vi "Monitornew new.vi"() -> ()   [LabVIEW 2019]
uses:
  <vilib>/Utility/file.llb/Write Delimited Spreadsheet (string).vi
  <userlib>/LevyLab/LV to ITX/Main/LV to DAT 1D.vi
panel:
  in  "shunt resistor":dbl=100000.0 format="%#_13g"
  in  "Tab Control":enum32{"Conductance"}(tab)
  in  "Voltage Pairs (+, -,...)":i32[][](array[numeric])=[[0, 0, 1, 2], [6, 6, 4, 3]]
  in  "Current (I-)":i32=3
  out "Two Terminal Conductance":cluster{"Y":dbl[], "Y":dbl[]}[](graph) caption="XY Graph"
  out "Four Terminal Resistance":cluster{"Y":dbl[], "Y":dbl[]}[](graph) caption="XY Graph"
  in  "Excitation voltage":dbl=0.1
  in  "Reset":bool
  out "Four Terminal conductance":cluster{"Y":dbl[], "Y":dbl[]}[](graph) caption="XY Graph"
  in  "wait (ms)":u32=60
  out "Humidity":dbl
  out "Temperature":dbl
  in  "error in (no error)":errorcluster
  in  "stop":bool
  in  "filename":string="test"
  in  "base path":path=path "G:/My Drive/ansom/Data/MFP3D/Test Files/monitor"
  in  "Comments":string
  in  "folder name":string="monitor"
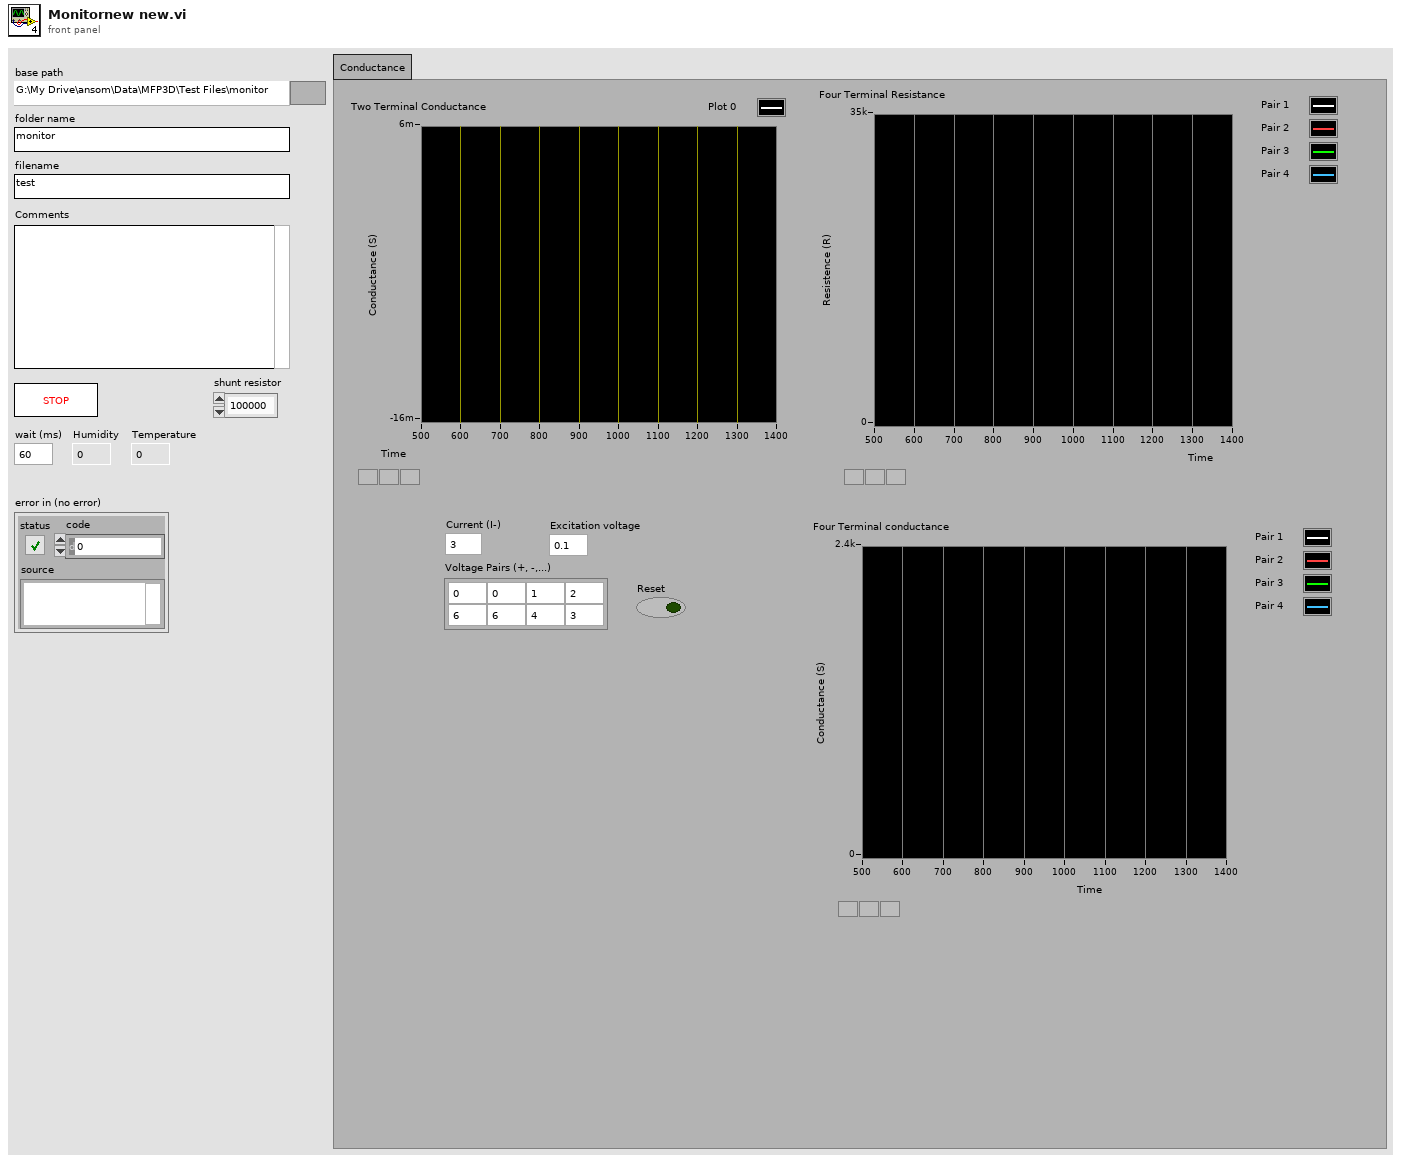
[diagram p1: front panel]
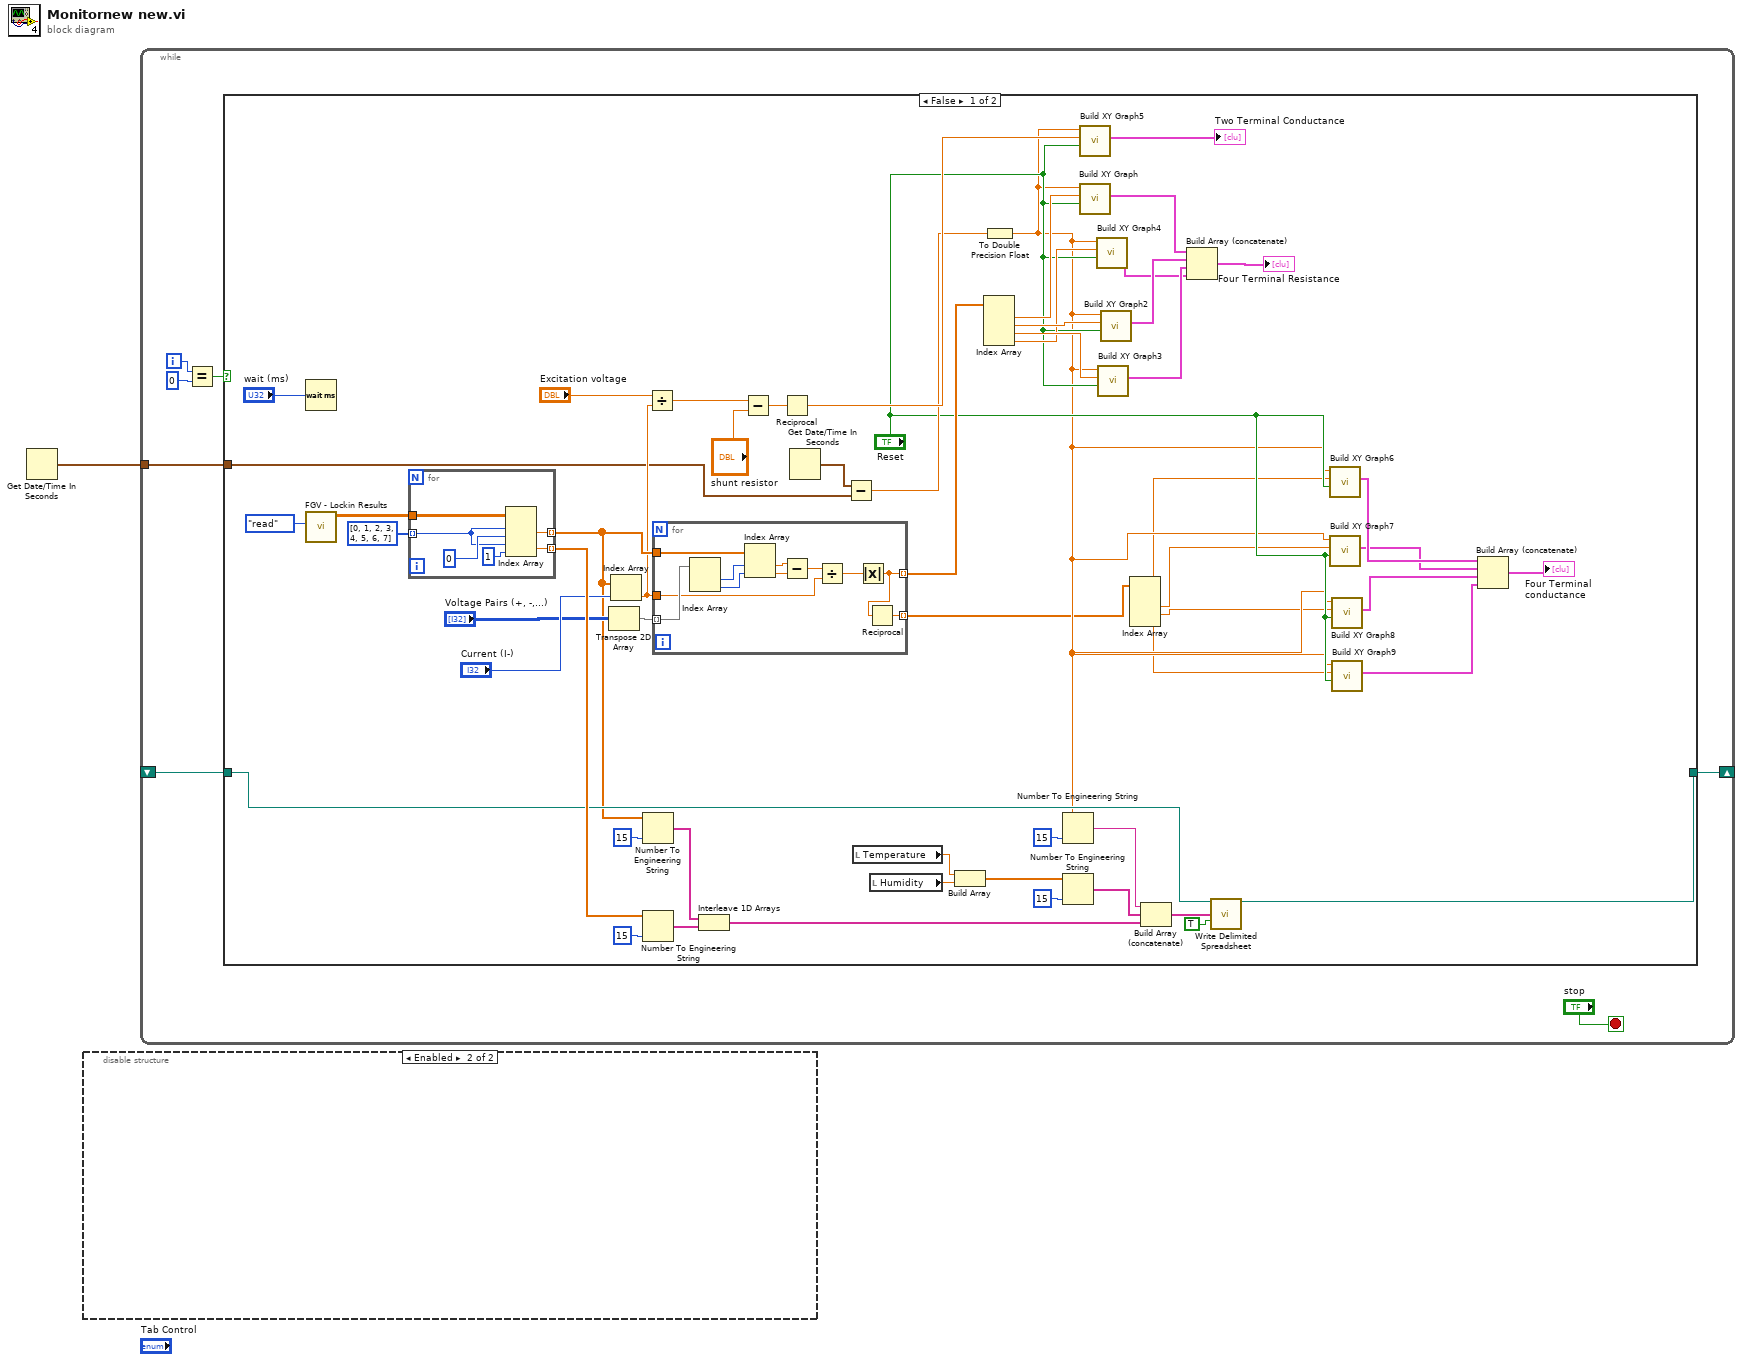
[diagram p0: block diagram]
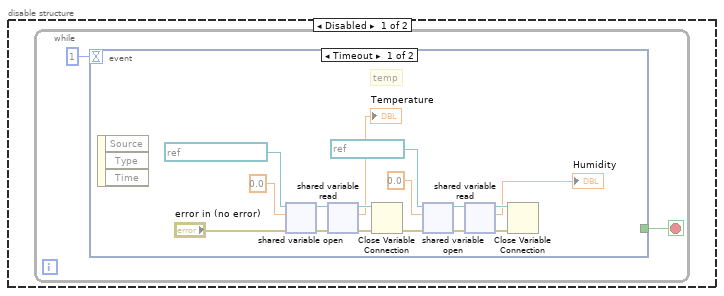
[diagram p2: hidden frame]
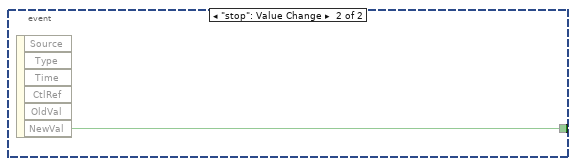
[diagram p3: hidden frame]
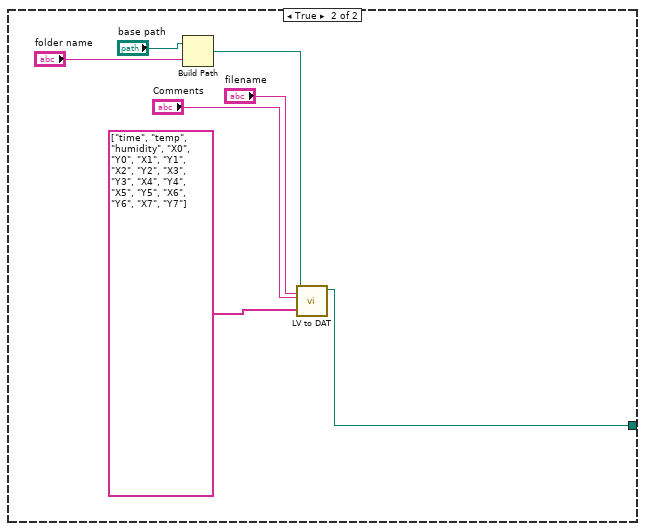
[diagram p4: hidden frame]
diagram:
  n1 = Get Date/Time In Seconds() -> (seconds since 1Jan1904=w1:timestamp)
  n2 = disable-structure shown="Enabled" {
    frame Disabled {
      n3 = while {
        stop <- w3 stop-if-true
        n4 = event shown="[0] Timeout" {
          selector: _ -> [_ _]
          dyn-events: _ -> [_ _]
          timeout: 1 -> [_ _]
          tunnel: [_ w20] -> w3
          event Timeout {
            # "temp"
            n5 = event-data() -> ()  [unwired: 1 in, 3 out]
            n6 = shared-variable-open(refnum<k21> "ni.var.psp://housesoftheholy/MFP3D/MFP3D Temperature" ("shared variable refnum in"), "error in (no error)", 0.0 ("Excitation voltage 2")) -> (w19:refnum<k21>, w18:errorcluster)  [unwired: 1 in]
            n7 = shared-variable-read(w19, w18) -> (w13:refnum<k21>, w12:errorcluster, →"Temperature":dbl)  [unwired: 1 out]
            n8 = Close Variable Connection(8:w12, 11:w13) -> (0:w6:errorcluster)
            n9 = shared-variable-open(refnum<k21> "ni.var.psp://housesoftheholy/MFP3D/MFP3D Hum" ("shared variable refnum in"), w6, 0.0 ("Excitation voltage 2")) -> (w16:refnum<k21>, w15:errorcluster)  [unwired: 1 in]
            n10 = shared-variable-read(w16, w15) -> (w11:refnum<k21>, w10:errorcluster, →"Humidity":dbl)  [unwired: 1 out]
            n11 = Close Variable Connection(8:w10, 11:w11) -> ()  [unwired: 1 out]
          }
          event "stop": Value Change {
            n12 = event-data() -> ("NewVal"=w20:bool)  [unwired: 1 in, 5 out]
          }
        }
      }
    }
    frame Enabled {
    }
  }
  n13 = while {
    shift-right: [w23] -> _
    shift-left: _ -> [w22]
    tunnel: w1 -> [w21]
    i -> [w27]
    stop <- "stop" stop-if-true
    n14 = Equal?(x=w27, y=0) -> (x = y?=w25:bool)
    n15 = case shown="False" w25 {
      tunnel: [w72 w102] -> w23
      tunnel: w22 -> [w75 _]
      tunnel: w21 -> [w48 _]
      frame False {
        n16 = Wait (ms)(milliseconds to wait="wait (ms)") -> ()  [unwired: 1 out]
        n17 = call <userlib>:"FGV - Lockin Results.vi"("Function"=enum16{"write", "read"}."read") -> ("Input Signals"=w82:dbl[][])  [unwired: 5 in, 1 out]
        n18 = for {
          tunnel: w82 -> [w98]
          tunnel: i32[] [0, 1, 2, 3, 4, 5, 6, 7] ("Lockins") -> [w99] mode=indexing
          tunnel: [w96] -> w60 mode=indexing
          tunnel: [w97] -> w76 mode=indexing
          n19 = Index Array(array=w98, index (row) #1=w99, index (col) #1=0 ("disabled index (col)"), index (row) #2=w99, index (col) #2=1 ("disabled index (col)")) -> (element #1=w96:dbl, element #2=w97:dbl)
        }
        n20 = Transpose 2D Array(2D array="Voltage Pairs (+, -,...)") -> (transposed array=w61:i32[][])
        n21 = Index Array(array=w60, index="Current (I-)") -> (element=w51:dbl)
        n22 = Number To Engineering String(2:i16 15 ("precision (6)"), 4:w60) -> (0:w79:string[])  [unwired: 2 out]
        n23 = Number To Engineering String(2:i16 15 ("precision (6)"), 4:w76) -> (0:w78:string[])  [unwired: 2 out]
        n24 = Divide(x="Excitation voltage", y=w51) -> (x/y=w45:dbl)
        n25 = for {
          tunnel: w61 -> [w95] mode=indexing
          tunnel: w60 -> [w94]
          tunnel: w51 -> [w89]
          tunnel: [w86] -> w59 mode=indexing
          tunnel: [w85] -> w32 mode=indexing
          n26 = Index Array(array=w95) -> (element #1=w93:i32, element #2=w92:i32)  [unwired: 2 in]
          n27 = Index Array(array=w94, index #1=w93, index #2=w92) -> (element #1=w91:dbl, element #2=w90:dbl)
          n28 = Subtract(x=w91, y=w90) -> (x-y=w88:dbl)
          n29 = Divide(x=w88, y=w89) -> (x/y=w87:dbl)
          n30 = Absolute Value(x=w87) -> (abs(x)=w86:dbl)
          n31 = Reciprocal(x=w86) -> (1/x=w85:dbl)
        }
        n32 = Interleave 1D Arrays(w79, w78) -> (w77:string[])
        n33 = Subtract(x=w45, y="shunt resistor") -> (x-y=w44:dbl)
        n34 = Reciprocal(x=w44) -> (1/x=w50:dbl)
        n35 = Get Date/Time In Seconds() -> (seconds since 1Jan1904=w49:timestamp)
        n36 = Subtract(x=w49, y=w48) -> (x-y=w47:dbl)
        n37 = local read "Temperature"() -> (w71:dbl)
        n38 = local read "Humidity"() -> (w70:dbl)
        n39 = Build Array(w71, w70) -> (w65:dbl[])
        n40 = Index Array(array=w59) -> (element #1=w58:dbl, element #2=w57:dbl, element #3=w56:dbl, element #4=w55:dbl)  [unwired: 4 in]
        n41 = To Double Precision Float(number=w47) -> (double precision float=w37:dbl)
        n42 = Number To Engineering String(2:i16 15 ("precision (6)"), 4:w37) -> (0:w67:string)  [unwired: 2 out]
        n43 = Number To Engineering String(2:i16 15 ("precision (6)"), 4:w65) -> (0:w64:string[])  [unwired: 2 out]
        n44 = call "Build XY Graph5"("Reset"="Reset", "Y Input"=w50, "X Input"=w37) -> ("XY Graph"=→"Two Terminal Conductance":cluster{"Y":dbl[], "Y":dbl[]}[])  [unwired: 2 in, 6 out]
        n45 = call "Build XY Graph"("Reset"="Reset", "Y Input"=w58, "X Input"=w37) -> ("XY Graph"=w54:cluster{"Y":dbl[], "Y":dbl[]}[])  [unwired: 2 in, 6 out]
        n46 = call "Build XY Graph4"("Reset"="Reset", "Y Input"=w55, "X Input"=w37) -> ("XY Graph"=w29:cluster{"Y":dbl[], "Y":dbl[]}[])  [unwired: 2 in, 6 out]
        n47 = call "Build XY Graph3"("Reset"="Reset", "Y Input"=w56, "X Input"=w37) -> ("XY Graph"=w30:cluster{"Y":dbl[], "Y":dbl[]}[])  [unwired: 2 in, 6 out]
        n48 = call "Build XY Graph2"("Reset"="Reset", "Y Input"=w57, "X Input"=w37) -> ("XY Graph"=w31:cluster{"Y":dbl[], "Y":dbl[]}[])  [unwired: 2 in, 6 out]
        n49 = Index Array(array=w32) -> (element #1=w36:dbl, element #2=w35:dbl, element #3=w34:dbl, element #4=w33:dbl)  [unwired: 4 in]
        n50 = Build Array (concatenate)(w67, w64, w77) -> (w73:string[])
        n51 = Build Array (concatenate)(w54, w31, w30, w29) -> (→"Four Terminal Resistance":cluster{"Y":dbl[], "Y":dbl[]}[])
        n52 = call-poly <vilib>:"Write Delimited Spreadsheet.vi"("file path (dialog if empty)"=w75, "1D data"=w73, "append to file? (new file:F)"=TRUE) -> ("new file path (Not A Path if cancelled)"=w72:path)  [unwired: 11 in, 1 out]
        n53 = call "Build XY Graph6"("Reset"="Reset", "Y Input"=w36, "X Input"=w37) -> ("XY Graph"=w43:cluster{"Y":dbl[], "Y":dbl[]}[])  [unwired: 2 in, 6 out]
        n54 = call "Build XY Graph7"("Reset"="Reset", "Y Input"=w35, "X Input"=w37) -> ("XY Graph"=w42:cluster{"Y":dbl[], "Y":dbl[]}[])  [unwired: 2 in, 6 out]
        n55 = call "Build XY Graph8"("Reset"="Reset", "Y Input"=w34, "X Input"=w37) -> ("XY Graph"=w41:cluster{"Y":dbl[], "Y":dbl[]}[])  [unwired: 2 in, 6 out]
        n56 = call "Build XY Graph9"("Reset"="Reset", "Y Input"=w33, "X Input"=w37) -> ("XY Graph"=w40:cluster{"Y":dbl[], "Y":dbl[]}[])  [unwired: 2 in, 6 out]
        n57 = Build Array (concatenate)(w43, w42, w41, w40) -> (→"Four Terminal conductance":cluster{"Y":dbl[], "Y":dbl[]}[])
      }
      frame True {
        n58 = Build Path(base path="base path", name or relative path="folder name") -> (appended path=w104:path)
        n59 = call-poly <userlib>:"LV to DAT.vi"("wavenames (.Vx, etc)"=string[] ["time", "temp", "humidity", "X0", "Y0", "X1", "Y1", "X2", "Y2", "X3", "Y3", "X4", "Y4", "X5", "Y5", "X6", "Y6", "X7", "Y7"], "filename"="filename", "Comments"="Comments", "path"=w104) -> ("new file path"=w102:path)  [unwired: 6 in, 1 out]
      }
    }
  }
